vi "PZT_oscillation.vi"() -> ()   [LabVIEW 2016]
panel:
  in  "PZT_oscillation":bool
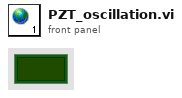
[diagram p1: front panel]
diagram:
